vi "node property program_0.vi"() -> ()   [LabVIEW 2015]
panel:
  in  "stop":bool
  in  "Tab Control":enum32{"Page 1", "Page 2"}(tab)
  in  "Numeric":dbl
  out "Blinking":bool
  # "Node property"
  # "Pardeep Kumar"
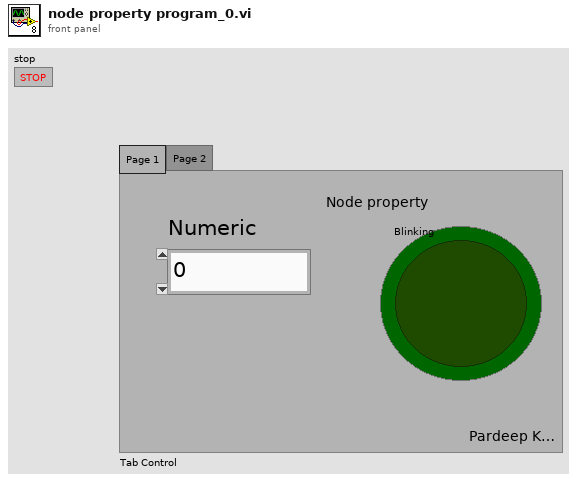
[diagram p1: front panel]
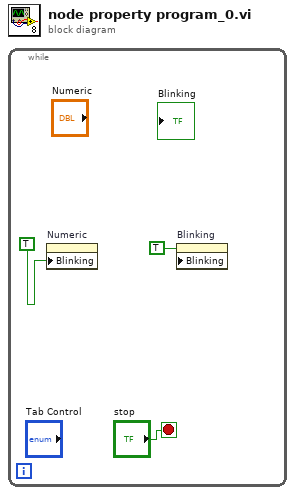
[diagram p0: block diagram]
diagram:
  n1 = while {
    stop <- "stop" stop-if-true
    n2 = property on="Numeric" class="DigNum (strict)"("Blinking"=TRUE) -> ()  [unwired: 2 in, 2 out]
    n3 = property on="Blinking" class="Bool (strict)"("Blinking"=TRUE) -> ()  [unwired: 2 in, 2 out]
  }
